vi "properties.to_json.vi"() -> ()   [LabVIEW 2020, in "type.lvclass"]
uses:
  type.lvclass
  properties.ctl
  property.ctl
  property value.ctl
  89e06e07-596b-4f08-8f01-ad3ba62158ca.vi
  <vilib>/JDP Science/JSONtext/Variant to JSON Text.vi
  <vilib>/JDP Science/JSONtext/LVClass Serializer/JSONtext LVClass Serializer.lvclass
  type.lvclass/type.ctl
  <vilib>/JDP Science/JSONtext/JSONtext.lvlib
panel:
  out "<JSON>":string caption="<JSON>First JSON Value"
  in  "properties":T1
  # "\"KeyName 2\": {\n      \"isRequired\": true,\n      \"description\": \"KeyDescription 2\"\n    }"
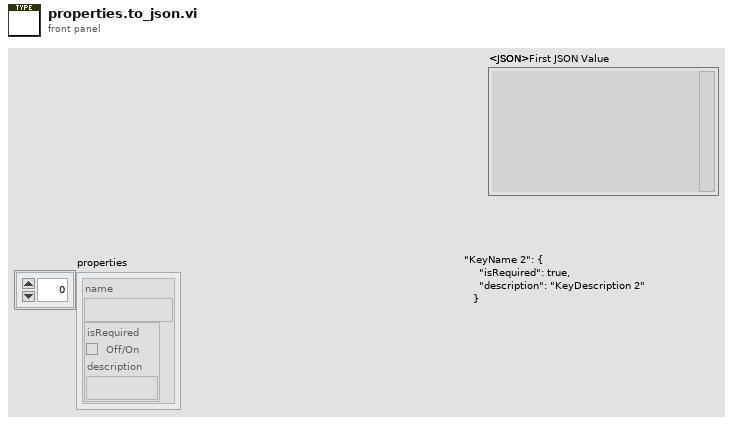
[diagram p1: front panel]
types:
  T1 = typedef "type.lvclass/properties.ctl" = T2[]
  T2 = typedef "type.lvclass/property.ctl" = cluster{"name":string, "value":T3}
  T3 = typedef "type.lvclass/property value.ctl" = cluster{"isRequired":bool, "description":string}
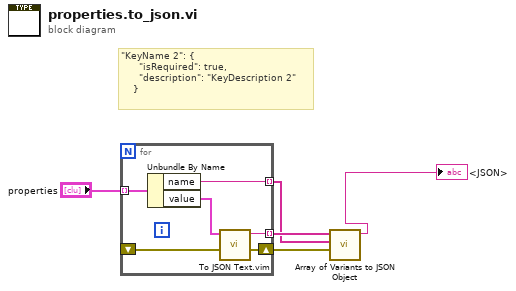
[diagram p0: block diagram]
diagram:
  # "\"KeyName 2\": {\n      \"isRequired\": true,\n      \"description\": \"KeyDescription 2\"\n    }"
  n1 = for {
    tunnel: "properties" -> [w11] mode=indexing
    tunnel: [w9] -> w4 mode=indexing
    tunnel: [w8] -> w3 mode=indexing
    shift-right: [w7] -> w2
    shift-left: _ -> [w6]
    n2 = Unbundle By Name(w11) -> ("name"=w8:string, "value"=w10:T3)
    n3 = call "To JSON Text.vim"("error in (no error)"=w6, "Anything"=w10) -> ("error out"=w7:errorcluster, "<JSON>"=w9:string)  [unwired: 8 in]
  }
  n4 = call <vilib>:"Array of Variants to JSON Object.vi"("error in (no error)"=w2, "Names"=w3, "Array"=w4) -> ("<JSON>"=→"<JSON>":string)  [unwired: 7 in, 1 out]
